vi "test report gen.vi"() -> ()   [LabVIEW 2016]
uses:
  activeXtest/activeXtest 2015 Folder/sonde cluster from excel.ctl
  Sonde Value Percent Tol.ctl
  <vilib>/Utility/NIReport.llb/NI_report.lvclass
panel:
  in  "Sonde Parameters \nInitial Values":T1 {"Salinity Initial" format="%_4f"; "Temp Initial" format="%_4f"; "ORP  Initial" format="%_2f"; "pH Initial" format="%_3f"; "DO Initial" format="%_3f"; "SC Initial" format="%_4f"}
  in  "Sonde Parameters \nTolerance Limits":T2 {"Salinity %" format="%_2f%%"; "Temp %" format="%_2f%%"; "ORP %" format="%_2f%%"; "pH %" format="%_2f%%"; "DO %" format="%_2f%%"; "SC %" format="%_2f%%"}
  out "actual number of rows":i32
  in  "error in":errorcluster
  out "error out 2":errorcluster
  out "Row":string[](array[string])
  out "Sonde Parameters Array":T3[](array[typedef]) {"Salinity"."%" format="%_2f%%"; "Salinity"."Value" format="%_4g"; "Temperature"."%" format="%_2f%%"; "Temperature"."Value" format="%_4g"; "ORP"."%" format="%_2f%%"; "ORP"."Value" format="%_4g"; "pH"."%" format="%_2f%%"; "pH"."Value" format="%_4g"; "Dissolved Oxygen"."%" format="%_2f%%"; "Dissolved Oxygen"."Value" format="%_4g"; "Sp. Conductance"."%" format="%_2f%%"; "Sp. Conductance"."Value" format="%_4g"; "Head" format="%#_4g"; "Cumulative\nVolume" format="%#_4g"}
  in  "report file path":path=path "D:/Cascade/templates/Groundwater Profiling Log_empty_2.xlsx"
  out "error out":errorcluster
  out "Sonde Data Array":string[][](array[string])
  out "row max value":i32
  out "Select Worksheet Index":i32
  out "Current Sample Sheet":string="Sample 1"
  out "start of Sample Sheets":i32
  in  "error in (no error)":errorcluster
  out "Worksheet Names":string[](array[string])
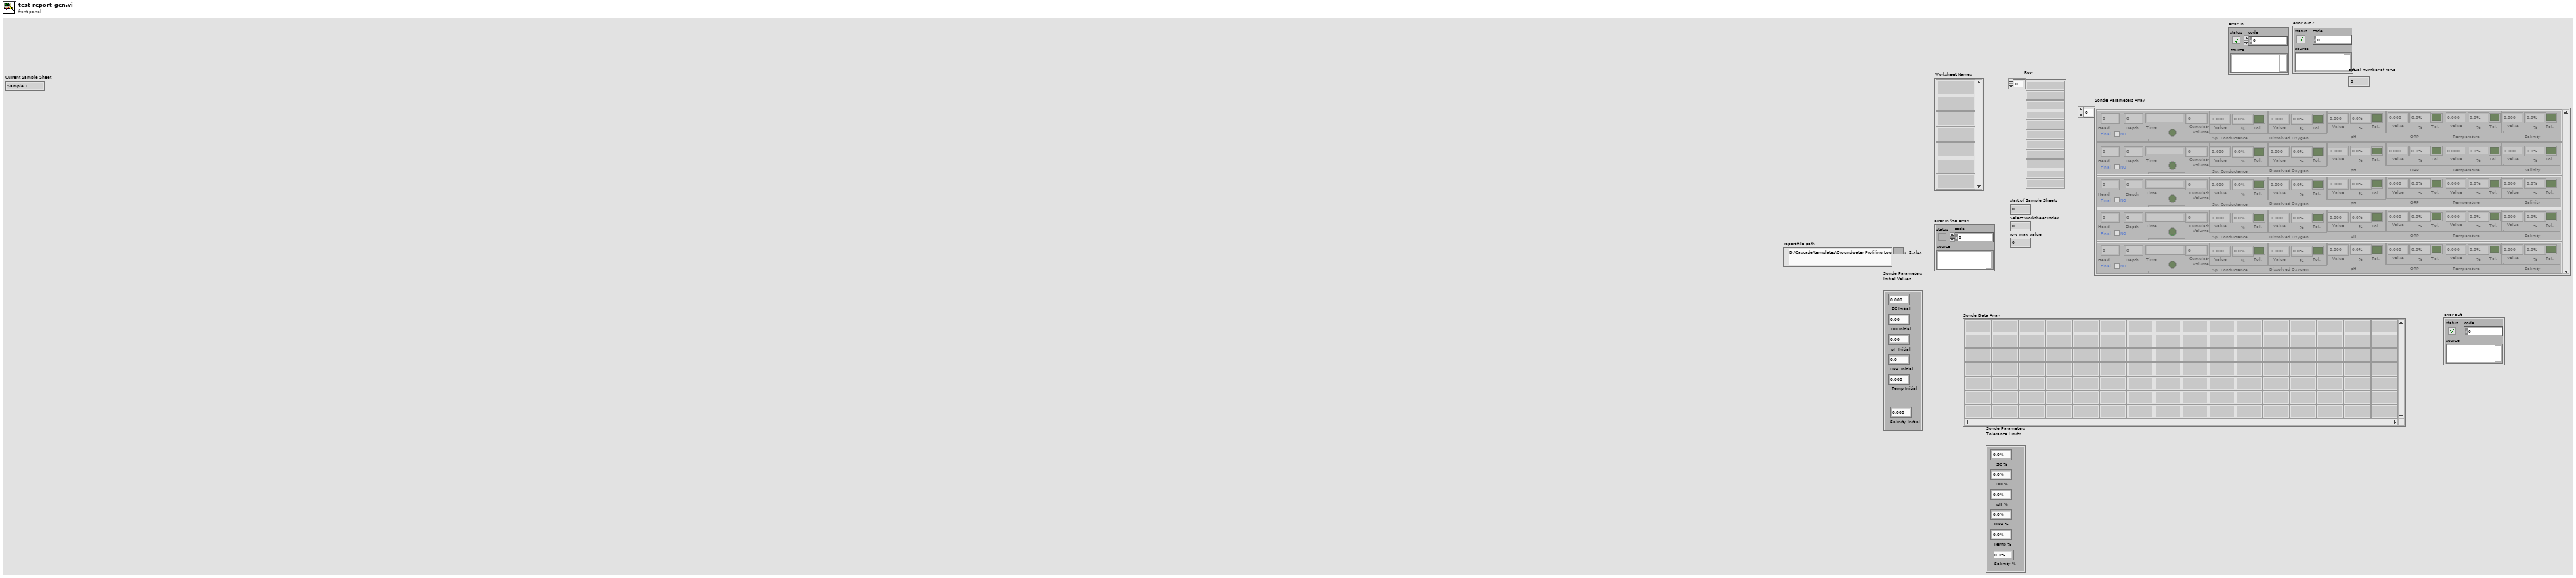
[diagram p1: front panel]
types:
  T1 = cluster{"SC Initial ":dbl, "DO Initial ":dbl, "pH Initial  ":dbl, "ORP  Initial":dbl, "Temp Initial":dbl, "Salinity Initial ":dbl}
  T2 = cluster{"SC %":dbl, "DO %":dbl, "pH % ":dbl, "ORP % ":dbl, "Temp % ":dbl, "Salinity %":dbl}
  T3 = typedef "sonde cluster from excel.ctl" = cluster{"Head":dbl, "Depth":dbl, "Time":string, "Cumulative\nVolume":dbl, "Sp. Conductance":T4, "Dissolved Oxygen":T4, "pH":T4, "ORP":T4, "Temperature":T4, "Salinity":T4, "Final Tol.":bool, "Final":bool, "Time 2":timestamp, "Aux 1":dbl, "Aux 2":dbl, "Aux 3":dbl}
  T4 = typedef "Sonde Value Percent Tol.ctl" = cluster{"Value":dbl, "%":dbl, "Tol.":bool}
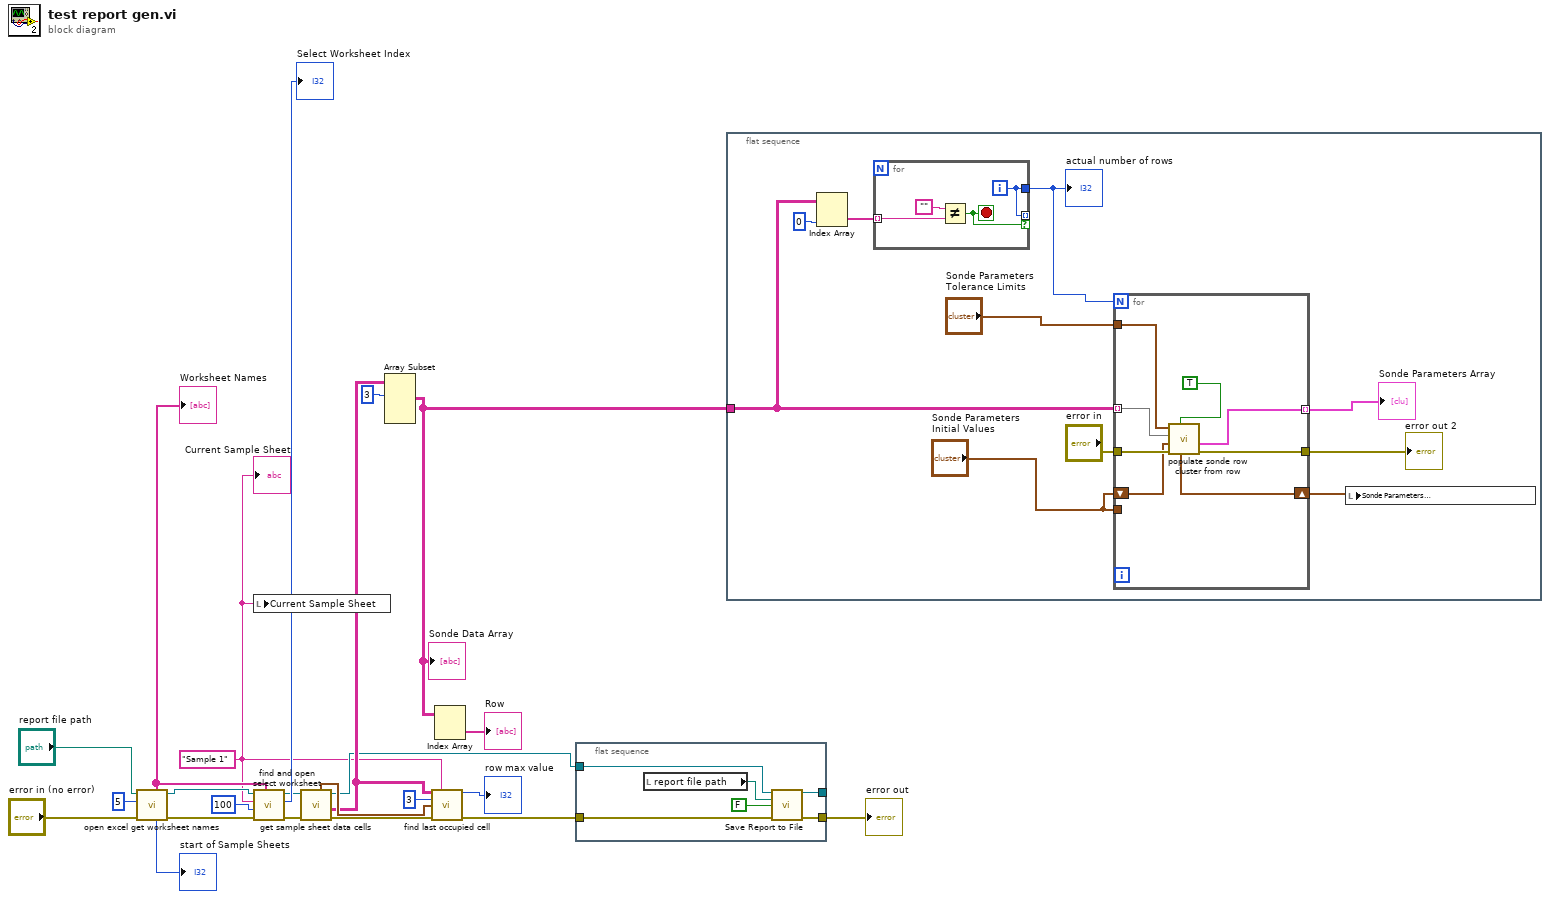
[diagram p0: block diagram]
diagram:
  w6 = "Sample 1" ("Worksheet Name in")
  n1 = call "open excel get worksheet names.vi"("error in (no error)"="error in (no error)", "milliseconds to wait"=u32 5, "report file path"="report file path") -> ("error out"=w19:errorcluster, "NI_report out"=w18:refnum<class "NI_report.lvclass">, "start of Sample Sheets"=→"start of Sample Sheets":i32, "Worksheet Names"=w17:string[])  [unwired: 3 in, 2 out]
  "Worksheet Names" <- w17
  n2 = local write "Current Sample Sheet"(w6) -> ()
  n3 = call "find and open select worksheet.vi"("Worksheet Names"=w17, "error in (no error)"=w19, "milliseconds to wait"=u32 100, "Worksheet Name in"=w6, "NI_report in"=w18) -> ("error out"=w12:errorcluster, "Select Worksheet Index"=→"Select Worksheet Index":i32, "NI_report out"=w11:refnum<class "NI_report.lvclass">)  [unwired: 4 in]
  n4 = call "get sample sheet data cells.vi"("error in (no error)"=w12, "NI_report in"=w11) -> ("error out"=w14:errorcluster, "data"=w10:string[][], "NI_report out"=w7:refnum<class "NI_report.lvclass">, "left edge output cluster"=w13:cluster{"row":i32, "column":i32})  [unwired: 5 in, 1 out]
  n5 = Array Subset(array=w10, index (row)=3 ("index")) -> (w1:string[][])  [unwired: 3 in]
  "Sonde Data Array" <- w1
  n6 = call "find last occupied cell.vi"("data"=w10, "Active Sheet"=w6, "Header Rows to remove"=3, "sub array start"=w13, "error in (no error)"=w14) -> ("row max value"=→"row max value":i32, "error out"=w8:errorcluster)  [unwired: 4 in, 5 out]
  n7 = Index Array(array=w1) -> (element=→"Row":string[])  [unwired: 2 in]
  n8 = flat-sequence {
    tunnel: [w29] -> _
    tunnel: [w28] -> w5
    tunnel: w8 -> [w26]
    tunnel: w7 -> [w25]
    frame #0 {
      n9 = local read "report file path"() -> (w24:path)
      n10 = call-dynamic "Save Report to File.vi"("report in"=w25, "report file path"=w24, "prompt to replace? (F)"=FALSE, "error in (no error)"=w26) -> ("report out"=w29:refnum<class "NI_report.lvclass">, "error out"=w28:errorcluster)  [unwired: 10 in]
    }
  }
  n11 = flat-sequence {
    tunnel: w1 -> [w34]
    frame #0 {
      n12 = Index Array(array=w34, index (col)=0 ("disabled index (col)")) -> (element=w35:string[])  [unwired: 1 in]
      n13 = for {
        tunnel: w35 -> [w43] mode=indexing
        tunnel: [w40] -> _ mode=indexing if=w41
        tunnel: [w40] -> w36
        i -> [w40]
        stop <- w41 stop-if-true
        n14 = Not Equal?(x="", y=w43) -> (x != y?=w41:bool)
      }
      "actual number of rows" <- w36
      n15 = for {
        N: w36 -> [_]
        tunnel: w34 -> [w50] mode=indexing
        tunnel: [w51] -> w39 mode=indexing
        tunnel: "error in" -> [w49]
        tunnel: "Sonde Parameters \nTolerance Limits" -> [w48]
        tunnel: "Sonde Parameters \nInitial Values" -> [_]
        shift-right: [w46] -> w31
        shift-left: "Sonde Parameters \nInitial Values" -> [w47]
        tunnel: [w44] -> w30
        n16 = call "populate sonde row cluster from row.vi"("Initialize Initial Value Cluster"=TRUE, "error in (no error)"=w49, "Sonde Parameters \nInitial Values"=w47, "Array In"=w50, "Sonde Parameters \nTolerance Limits"=w48) -> ("error out"=w44:errorcluster, "Cluster"=w51:T3, "Sonde Parameters \nInitial Values Out"=w46:T1)  [unwired: 3 in, 1 out]
      }
      "Sonde Parameters Array" <- w39
      "error out 2" <- w30
      n17 = local write "Sonde Parameters \nInitial Values"(w31) -> ()
    }
  }
  "Current Sample Sheet" <- w6
  "error out" <- w5
